vi "log_data.vi"(8 "error in (no error)":errorcluster, 9 "Test":T1, 10 "Elements Remaining":u32, 11 "Data":fxp<+/-,24,4>[](array[numeric])) -> (0 "error out":errorcluster, 2 "Ref file Data out":refnum<file>[](array[refnum]), 3 "Number of elements out":u32)   [LabVIEW 2015]
uses:
  controls/Test Data.ctl
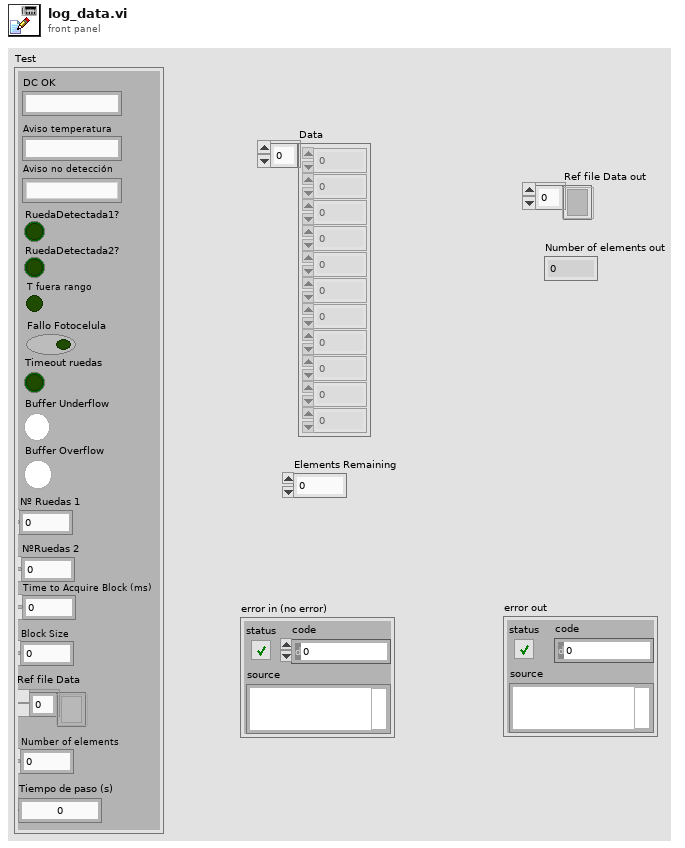
[diagram p1: front panel]
types:
  T1 = typedef "Test Data.ctl" = cluster{"DC OK":string, "Aviso temperatura":string, "Aviso no detección":string, "RuedaDetectada1?":bool, "RuedaDetectada2?":bool, "T fuera rango":bool, "Fallo Fotocelula":bool, "Timeout ruedas":bool, "Buffer Underflow":bool, "Buffer Overflow":bool, "Nº Ruedas 1":i32, "NºRuedas 2":i32, "Block Size":u32, "Time to Acquire Block (ms)":i32, "Ref file Data":refnum<file>[], "Number of elements":u32, "Tiempo de paso (s)":dbl}
  T2 = enum16{"big-endian, network order", "native, host order", "little-endian"}
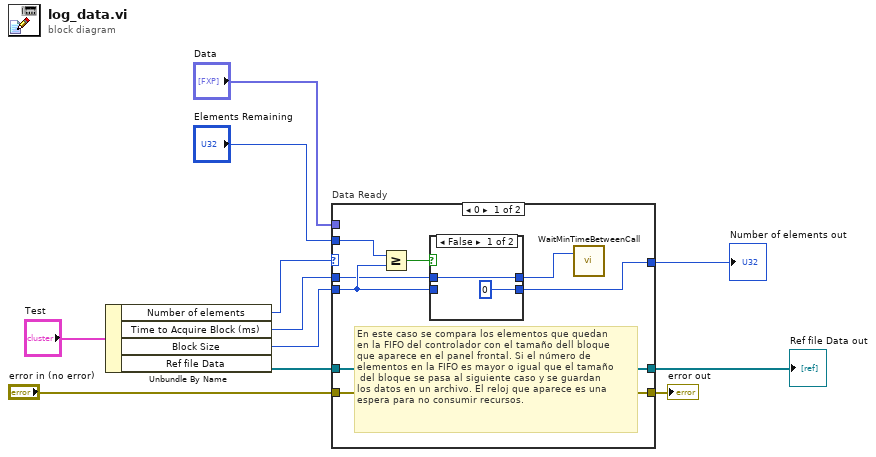
[diagram p0: block diagram]
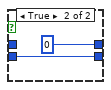
[diagram p2: hidden frame]
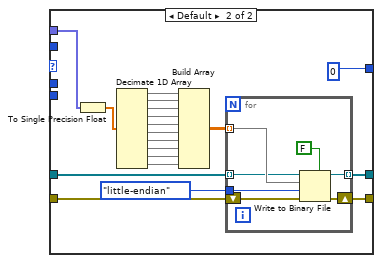
[diagram p3: hidden frame]
diagram:
  n1 = Unbundle By Name("Test") -> ("Number of elements"=w7:u32, "Time to Acquire Block (ms)"=w5:i32, "Block Size"=w6:u32, "Ref file Data"=w4:refnum<file>[])
  n2 = case "Data Ready" shown="0" w7 {
    tunnel: w5 -> [w16 _]
    tunnel: [w15 u32 0 ("t")] -> w10
    tunnel: w6 -> [w17 _]
    tunnel: "Elements Remaining" -> [w14 _]
    tunnel: "Data" -> [_ w39]
    tunnel: "error in (no error)" -> [w13 w38]
    tunnel: [w13 w40] -> w1
    tunnel: w4 -> [w12 w37]
    tunnel: [w12 w36] -> w9
    frame 0 {
      # "En este caso se compara los elementos que quedan\nen la FIFO del controlador con el tamaño dell bloque\nque aparece en el panel frontal. Si el número de \nelementos en la FIFO es mayor o igual que el tamaño\n del bloque se pasa al siguiente caso y se guardan \nlos datos en un archivo. El reloj que aparece es una\nespera para no consumir recursos."
      n3 = Greater Or Equal?(x=w14, y=w17) -> (x >= y?=w18:bool)
      n4 = case shown="False" w18 {
        tunnel: [u32 0 ("Block Size") w22] -> w15
        tunnel: [w21 0 ("t")] -> w19
        tunnel: w16 -> [w21 _]
        tunnel: w17 -> [_ w22]
        frame False {
        }
        frame True {
        }
      }
      n5 = call "WaitMinTimeBetweenCall.vi"("Minimum ms between calls"=w19) -> ()  [unwired: 2 in]
    }
    frame Default {
      n6 = To Single Precision Float(number=w39) -> (single precision float=w26:sgl[])
      n7 = Decimate 1D Array(w26) -> (w32:sgl[], w35:sgl[], w34:sgl[], w33:sgl[], w31:sgl[], w30:sgl[], w29:sgl[], w28:sgl[], w27:sgl[], w24:sgl[])
      n8 = Build Array(w32, w35, w34, w33, w31, w30, w29, w28, w27, w24) -> (w25:sgl[][])
      n9 = for {
        tunnel: T2."little-endian" ("byte order (0:big-endian, network order)") -> [w49]
        shift-right: [w43] -> w40
        shift-left: w38 -> [w44]
        tunnel: w25 -> [w47] mode=indexing
        tunnel: w37 -> [w46] mode=indexing
        tunnel: [w45] -> w36 mode=indexing
        n10 = Write to Binary File(file (use dialog)=w46, data=w47, error in=w44, 5:FALSE ("prepend array or string size? (T)"), 9:w49) -> (refnum out=w45:refnum<file>, error out=w43:errorcluster)  [unwired: 2 out]
      }
    }
  }
  "Number of elements out" <- w10
  "Ref file Data out" <- w9
  "error out" <- w1
